vi "sort module schedule.vi"(11 "priority array":T1(array[cluster])) -> (3 "sorted module indices":i32[](array[numeric]))   [LabVIEW 2013, in "Standard Engine Runtime.lvclass"]
uses:
  Standard Engine Runtime.lvclass
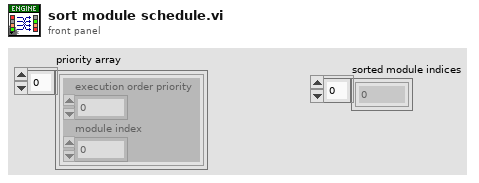
[diagram p1: front panel]
types:
  T1 = cluster{"execution order priority":i32, "module index":i32}[]
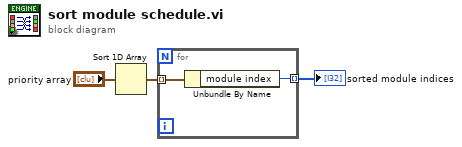
[diagram p0: block diagram]
diagram:
  n1 = Sort 1D Array(array="priority array") -> (sorted array=w2:T1)
  n2 = for {
    tunnel: w2 -> [w5] mode=indexing
    tunnel: [w4] -> w1 mode=indexing
    n3 = Unbundle By Name(w5) -> ("module index"=w4:i32)
  }
  "sorted module indices" <- w1
